vi "Drive Straight Profiled PID.vi"(4 "Gyro PIDF":cluster{"Kp":dbl, "Ki":dbl, "Kd":dbl, "Kf":dbl}={"Kp"=0.05, "Ki"=0.0, "Kd"=0.0, "Kf"=0.0} {"Kf" format="%.3f"; "Kd" format="%.3f"; "Ki" format="%.3f"; "Kp" format="%.3f"}, 5 "Angle Offset":dbl, 6 "Iteration":i32, 7 "Position Tolerance":dbl format="%#_13g", 8 "dt (s)":dbl=10.0, 9 "target distance":dbl, 10 "Odometry":T1, 11 "PID Ref in":refnum<data-value>) -> (1 "At Target?":bool, 2 "Right Speed":dbl, 3 "Left Speed":dbl)   [LabVIEW 2019]
uses:
  Odometry/Typedef/Odometry.ctl
  <vilib>/Rock Robotics/WPI/ThirdParty/WPILib Extensions/Geometry/Typedef/Pose2d.ctl
  <vilib>/Rock Robotics/WPI/ThirdParty/WPILib Extensions/Geometry/Typedef/Translation2d.ctl
  <vilib>/Rock Robotics/WPI/ThirdParty/WPILib Extensions/Geometry/Typedef/Rotation2d.ctl
  <vilib>/Rock Robotics/WPI/ThirdParty/WPILib Extensions/Controller/PID/Typedef/PID Controller State.ctl
panel:
  out "Waveform Chart 3":cluster{"Position":dbl, "Velocity":dbl}(graph)
  out "Waveform Chart 2":cluster{dbl, dbl}(graph)={-50.0, -50.00778875}
  out "Gyro Output":dbl(graph)=0.02713616249999992
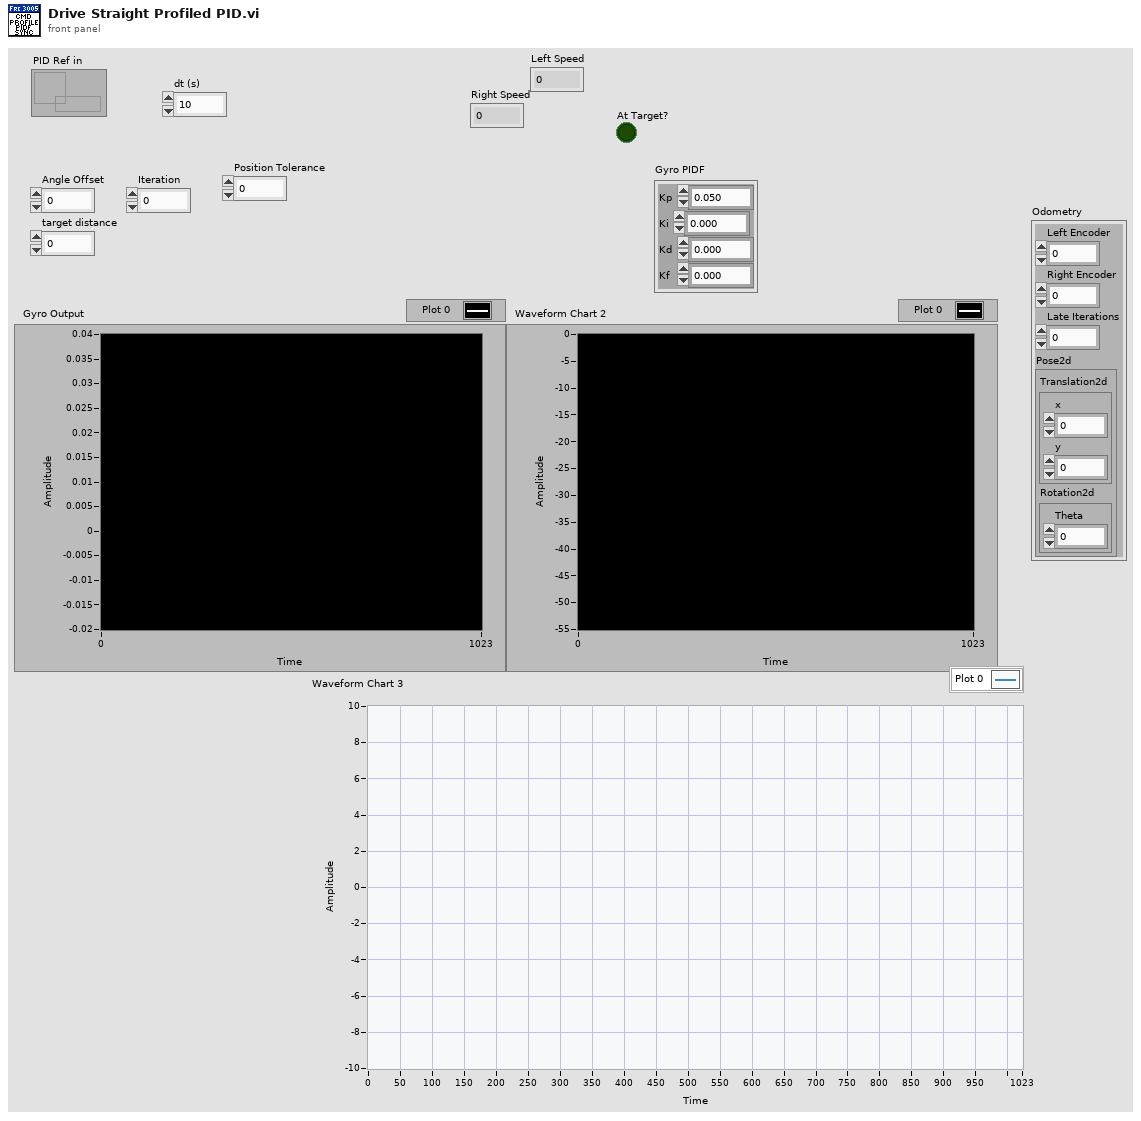
[diagram p1: front panel]
types:
  T1 = typedef "Odometry.ctl" = cluster{"Left Encoder":dbl, "Right Encoder":dbl, "Late Iterations":u32, "Pose2d":T2}
  T2 = typedef "Pose2d.ctl" = cluster{"Translation2d":T3, "Rotation2d":T4}
  T3 = typedef "Translation2d.ctl" = cluster{"x":dbl, "y":dbl}
  T4 = typedef "Rotation2d.ctl" = cluster{"Theta":dbl}
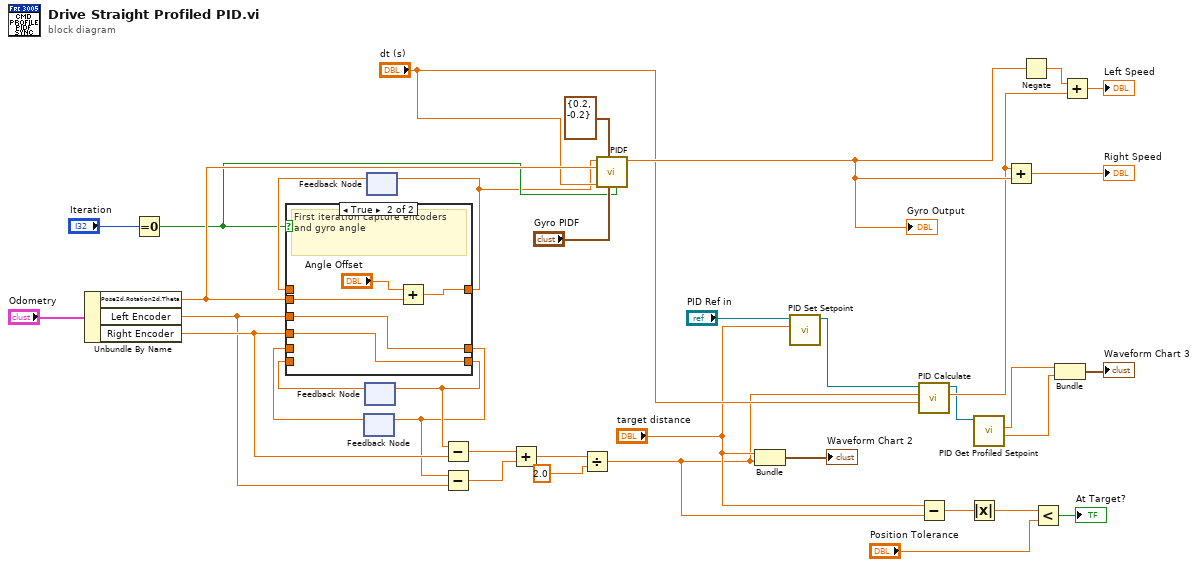
[diagram p0: block diagram]
diagram:
  n1 = Unbundle By Name("Odometry") -> ("Pose2d.Rotation2d.Theta"=w19:dbl, "Left Encoder"=w23:dbl, "Right Encoder"=w25:dbl)
  n2 = Equal To 0?(x="Iteration") -> (x = 0?=w16:bool)
  n3 = feedback #1() -> (w27:dbl)  [unwired: 1 in]
  n4 = feedback #2() -> (w28:dbl)  [unwired: 1 in]
  n5 = feedback #3() -> (w32:dbl)  [unwired: 1 in]
  n6 = case shown="True" w16 {
    tunnel: [w40 w44] -> w12
    tunnel: w32 -> [w40 _]
    tunnel: w19 -> [_ w43]
    tunnel: w23 -> [_ w41]
    tunnel: w25 -> [_ w42]
    tunnel: [w39 w42] -> w26
    tunnel: [w38 w41] -> w24
    tunnel: w28 -> [w39 _]
    tunnel: w27 -> [w38 _]
    frame False {
    }
    frame True {
      # "First iteration capture encoders and gyro angle"
      n7 = Add(x="Angle Offset", y=w43) -> (x+y=w44:dbl)
    }
  }
  n8 = feedback-in #1(w24) -> ()
  n9 = feedback-in #2(w26) -> ()
  n10 = feedback-in #3(w12) -> ()
  n11 = Subtract(x=w26, y=w25) -> (x-y=w22:dbl)
  n12 = Subtract(x=w24, y=w23) -> (x-y=w21:dbl)
  n13 = Add(x=w22, y=w21) -> (x+y=w37:dbl)
  n14 = Divide(x=w37, y=2.0) -> (x/y=w9:dbl)
  n15 = call <vilib>:"PIDF.vi"("reinitialize? (F)"=w16, "PIDF gains"="Gyro PIDF", "output range"=cluster{"output high":dbl, "output low":dbl} {"output high"=0.2, "output low"=-0.2}, "dt (s)"="dt (s)", "process variable"=w19, "setpoint"=w12) -> ("output"=w18:dbl)  [unwired: 3 in, 2 out]
  "Gyro Output" <- w18
  n16 = Bundle("target distance"="target distance", w9) -> (→"Waveform Chart 2":cluster{"target distance":dbl, dbl})  [unwired: 1 in]
  n17 = call <vilib>:"PID Set Setpoint.vi"("Setpoint"="target distance", "PID Ref"="PID Ref in") -> ("PID Ref"=w13:refnum<data-value>)  [unwired: 9 in]
  n18 = call <vilib>:"PID Calculate.vi"("dt (s)"="dt (s)", "Process Variable"=w9, "PID Ref in"=w13) -> ("output"=w11:dbl, "PID Ref out"=w3:refnum<data-value>)  [unwired: 7 in]
  n19 = Subtract(x="target distance", y=w9) -> (x-y=w8:dbl)
  n20 = Absolute Value(x=w8) -> (abs(x)=w7:dbl)
  n21 = call <vilib>:"PID Get Profiled Setpoint.vi"("Data Value Reference in"=w3) -> ("Velocity"=w1:dbl, "Position"=w2:dbl)  [unwired: 8 in, 1 out]
  n22 = Add(x=w11, y=w18) -> (x+y=→"Right Speed":dbl)
  n23 = Negate(x=w18) -> (-x=w34:dbl)
  n24 = Less?(x=w7, y="Position Tolerance") -> (x < y?=→"At Target?":bool)
  n25 = Bundle("Position"=w2, "Velocity"=w1) -> (→"Waveform Chart 3":cluster{"Position":dbl, "Velocity":dbl})  [unwired: 1 in]
  n26 = Add(x=w34, y=w11) -> (x+y=→"Left Speed":dbl)
